vi "Swap Indices.vi"(8 "error in (no error)":errorcluster, 9 "Index B":i32, 10 "Index A":i32, 11 "PanelArray in":refnum<class "ArrayManager.lvclass">) -> (0 "error out":errorcluster, 3 "PanelArray out":refnum<class "ArrayManager.lvclass">)   [LabVIEW 2020, in "OOPanel.lvlib" / "ArrayManager.lvclass"]
uses:
  <vilib>/IlluminatedG/IG OOPanel/OOPanel/ArrayManager/ArrayManager.lvclass
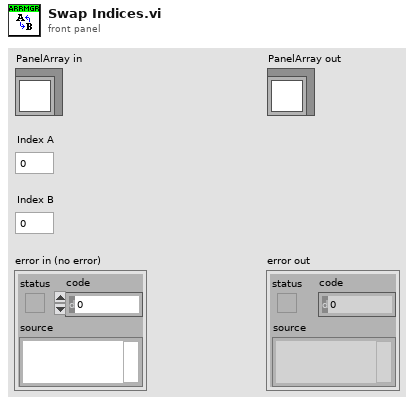
[diagram p1: front panel]
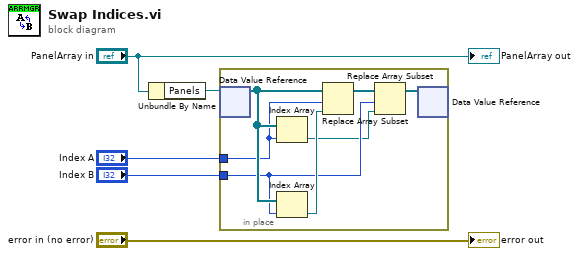
[diagram p0: block diagram]
diagram:
  n1 = Unbundle By Name("PanelArray in") -> ("Panels"=w4:refnum<data-value>)
  n2 = in-place {
    in-place-border: "Index A" -> [w10]
    in-place-border: "Index B" -> [w8]
    n3 = in-place-dvr #1(w4) -> (w12:refnum<class "ArrayPanel.lvclass">[])  [unwired: 1 out]
    n4 = Index Array(array=w12, index=w10) -> (element=w7:refnum<class "ArrayPanel.lvclass">)
    n5 = Index Array(array=w12, index=w8) -> (element=w11:refnum<class "ArrayPanel.lvclass">)
    n6 = Replace Array Subset(array=w12, new element=w11, index=w10) -> (w9:refnum<class "ArrayPanel.lvclass">[])
    n7 = Replace Array Subset(array=w9, new element=w7, index=w8) -> (w6:refnum<class "ArrayPanel.lvclass">[])
    n8 = in-place-dvr #1(w6) -> ()  [unwired: 2 out]
  }
  "error out" <- "error in (no error)"
  "PanelArray out" <- "PanelArray in"
